vi "Find Systems.vi"(4 "Only Installable Systems (F)":bool, 5 "Device Class":string, 6 "Timeout (4000 ms)":u32=4000, 7 "Detect Online Systems (T)":bool=TRUE, 8 "error in (no error)":errorcluster, 9 "Output (Hostname and IP)":u32(ring)=18 items=["Hostname"=16, "Hostname (IP)"=18, "Hostname (MAC)"=19, "IP"=32, "IP (Hostname)"=33, "IP (MAC)"=35, "MAC"=48, "MAC (Hostname)"=49, "MAC (IP)"=50], 10 "Include Cached Results (all)":u32(ring)=3 items=["none"=0, "only if online"=1, "all"=3], 11 "Session in (localhost)":refnum<k21>="localhost") -> (0 "error out":errorcluster, 2 "Detected Systems":string[](array[string]), 3 "Session out":refnum<k21>)   [LabVIEW 2012, in "nisyscfg.lvlib"]
doc: "Retrieves a list of systems on the network."
uses:
  <vilib>/nisyscfg/nisyscfg.lvlib
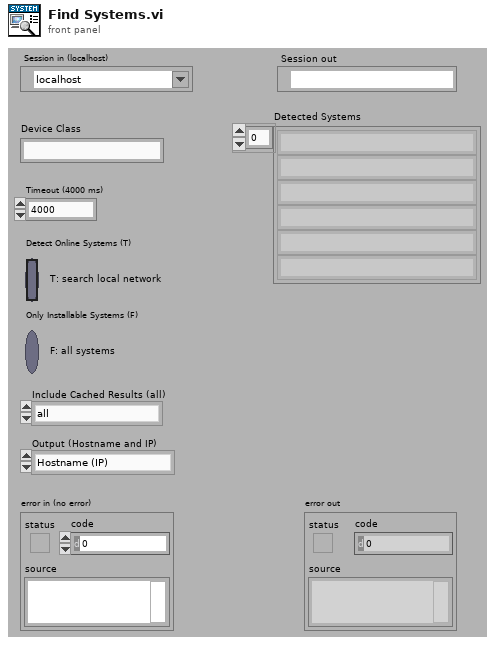
[diagram p1: front panel]
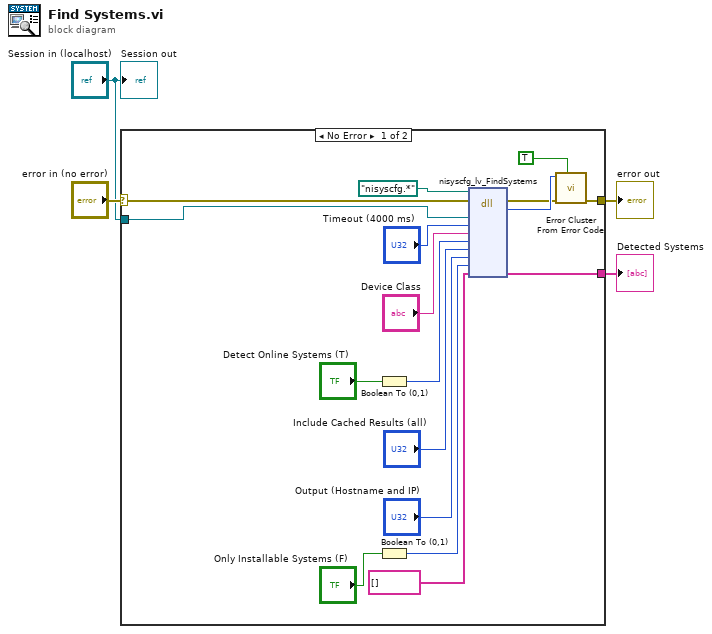
[diagram p0: block diagram]
diagram:
  n1 = case shown="No Error" "error in (no error)" {
    selector: "error in (no error)" -> [w19 w22]
    tunnel: [w9 w22] -> w4
    tunnel: [w11 _] -> w2
    tunnel: "Session in (localhost)" -> [w7 _]
    frame No Error {
      n2 = Boolean To (0,1)(Boolean="Detect Online Systems (T)") -> (0, 1=w13:i16)
      n3 = Boolean To (0,1)(Boolean="Only Installable Systems (F)") -> (0, 1=w5:i16)
      n4 = dll-call lib="nisyscfg.*" fn="nisyscfg_lv_FindSystems" label="FindSystems"(path in=path "nisyscfg.*", error in=w19, "session"=w7, "timeoutMsec"="Timeout (4000 ms)", "deviceClass"="Device Class", "doBroadcast"=w13, "cachedOptions"="Include Cached Results (all)", "outputFormat"="Output (Hostname and IP)", "onlyInstallableSystems"=w5, "systems"=string[] [] ("Array")) -> (error out=w20:errorcluster, "result"=w21:i32, "systems"=w11:string[])  [unwired: 8 in, 1 out]
      n5 = call <vilib>:"Error Cluster From Error Code.vi"("show call chain? (False)"=TRUE, "error in (no error)"=w20, "error code (0)"=w21) -> ("error out"=w9:errorcluster)  [unwired: 6 in]
    }
    frame Error {
    }
  }
  "error out" <- w4
  "Detected Systems" <- w2
  "Session out" <- "Session in (localhost)"
